vi "Save Settings to XML.vi"(8 "error in (no error)":errorcluster, 11 "Settings":T1={"Hardware Configuration"={"AVS Settings"={"Communication Settings"={"Serial1"="", "Handle1"=0, "a_pDeviceId1"=[], "a_pNumPixels"=0, "Port"=0, "a_hWnd"=0}, "a_pMeasConfig1"={"StartPixel"=0, "StopPixel"=0, "IntTime"=0.0, "IntDelay"=0, "NrOfAVG"=0, "DarkEnable"=0, "ForgetPercentage"=0, "SmoothPix"=0, "SmoothModel"=0, "SatDetection"=0, "TriggerMode"=0, "TriggerSource"=0, "TriggerSourceType"=0, "FlashesPerScan"=0, "LaserDelay"=0, "LaserWidth"=0, "LaserWavelenght"=0.0, "RamSpectra"=0}, "Dark Correct"=TRUE, "Auto Determine Int Time"=TRUE}, "Sphere Indicator"=enum."Naked Sphere", "Measurement Type"=enum."Normal", "Correction Files"={"Calibration File"=path "", "Cal lamp in, cal lamp on"=path "", "Cal lamp in, aux lamp on"=path "", "DUT in, aux lamp on"=path "", "Dark Array Model"=path ""}}, "Logging Configuration"={"Log File Base Path"=path "", "Cal File Folder"=path "", "TDMS File Reference"=refnum}, "Base Path"=path ""}) -> (0 "error out":errorcluster)   [LabVIEW 2013, in "AvaSpec.lvlib" / "AvaSpec Settings.lvlib"]
doc: "Saves the \"User Specified\" configuration data to an XML file. This is used to remember the users settings between executions."
uses:
  AvaSpec Settings.lvlib
  Settings.ctl
  Acquisition/Hardware Configuration.ctl
  Libraries/AS-5216-DLL/AVS settings.ctl
  Acquisition/Sphere Indicator.ctl
  Measurement Type.ctl
  Logging/Logging Configuration.ctl
  <vilib>/Utility/xml.llb/Write to XML File(string).vi
  Acquisition/AvaSpec Acquisition.lvlib
  Logging/AvaSpec Logging.lvlib
  AvaSpec.lvlib
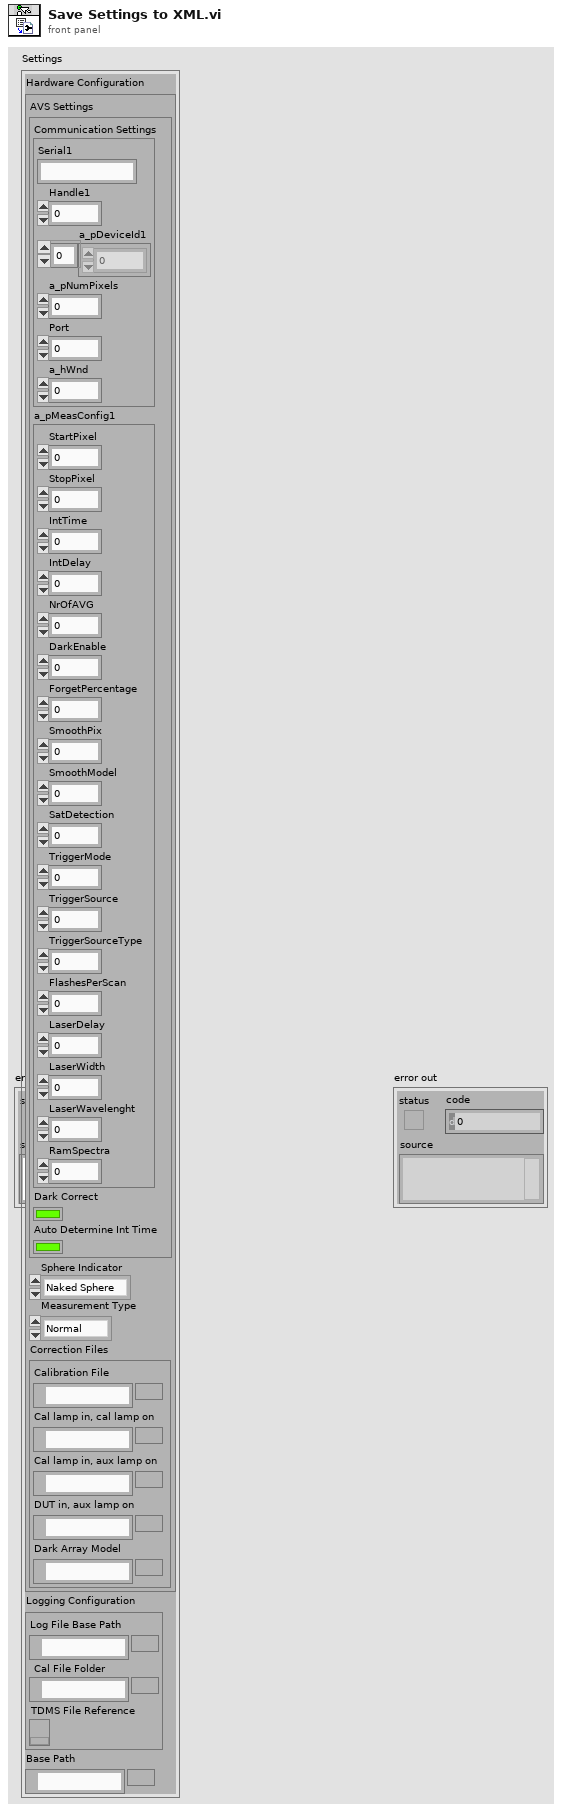
[diagram p1: front panel]
types:
  T1 = typedef "AvaSpec.lvlib/AvaSpec Settings.lvlib/Settings.ctl" = cluster{"Hardware Configuration":T2, "Logging Configuration":T6, "Base Path":path}
  T2 = typedef "AvaSpec.lvlib/AvaSpec Acquisition.lvlib/Hardware Configuration.ctl" = cluster{"AVS Settings":T3, "Sphere Indicator":T4, "Measurement Type":T5, "Correction Files":cluster{"Calibration File":path, "Cal lamp in, cal lamp on":path, "Cal lamp in, aux lamp on":path, "DUT in, aux lamp on":path, "Dark Array Model":path}}
  T3 = typedef "AvaSpec.lvlib/AVS settings.ctl" = cluster{"Communication Settings":cluster{"Serial1":string, "Handle1":i32, "a_pDeviceId1":u8[], "a_pNumPixels":u16, "Port":i32, "a_hWnd":i32}, "a_pMeasConfig1":cluster{"StartPixel":u16, "StopPixel":u16, "IntTime":sgl, "IntDelay":u32, "NrOfAVG":u32, "DarkEnable":u8, "ForgetPercentage":u8, "SmoothPix":u16, "SmoothModel":u8, "SatDetection":u8, "TriggerMode":u8, "TriggerSource":u8, "TriggerSourceType":u8, "FlashesPerScan":u16, "LaserDelay":u32, "LaserWidth":u32, "LaserWavelenght":sgl, "RamSpectra":u16}, "Dark Correct":bool, "Auto Determine Int Time":bool}
  T4 = typedef "AvaSpec.lvlib/Sphere Indicator.ctl" = enum16{"Naked Sphere", "Insulated Sphere"}
  T5 = typedef "Measurement Type.ctl" = enum16{"Normal", "Calibration", "Dark"}
  T6 = typedef "AvaSpec.lvlib/AvaSpec Logging.lvlib/Logging Configuration.ctl" = cluster{"Log File Base Path":path, "Cal File Folder":path, "TDMS File Reference":refnum<k34>}
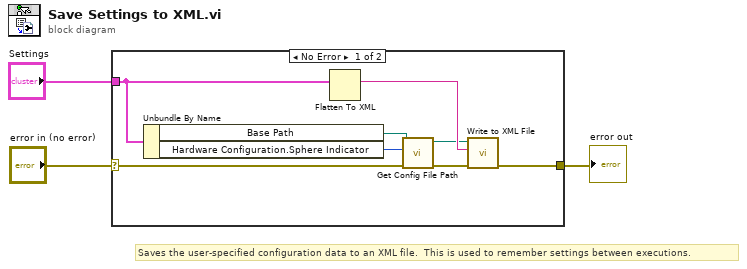
[diagram p0: block diagram]
diagram:
  # "Saves the user-specified configuration data to an XML file.  This is used to remember settings between executions."
  n1 = case shown="No Error" "error in (no error)" {
    selector: "error in (no error)" -> [w8 w12]
    tunnel: [w10 w12] -> w2
    tunnel: "Settings" -> [w6 _]
    frame No Error {
      n2 = Unbundle By Name(w6) -> ("Base Path"=w5:path, "Hardware Configuration.Sphere Indicator"=w4:T4)
      n3 = Flatten To XML(anything=w6) -> (xml string=w11:string)
      n4 = call "Get Config File Path.vi"("error in (no error)"=w8, "Sphere indicator"=w4, "Base Path"=w5) -> ("error out"=w7:errorcluster, "XML File Path"=w9:path)  [unwired: 6 in, 1 out]
      n5 = call-poly <vilib>:"Write to XML File.vi"("error in (no error)"=w7, "XML Input"=w11, "XML File Path"=w9) -> ("error out"=w10:errorcluster)  [unwired: 6 in, 2 out]
    }
    frame Error {
    }
  }
  "error out" <- w2
